vi "Nodos_Propiedad_Act02.vi"() -> ()   [LabVIEW 2020]
panel:
  in  "stop":bool
  out "String":string
  out "No. Muestreos":i32
  in  "Límite Muestreo":i32
  in  "Límite superior":dbl
  in  "Tiempo de muestreo":dbl
  out "Fuera de rango":bool
  out "Temperatura":cluster{dbl, "Límite superior":dbl}(graph)
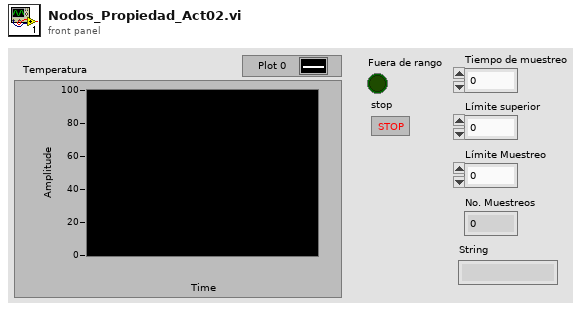
[diagram p1: front panel]
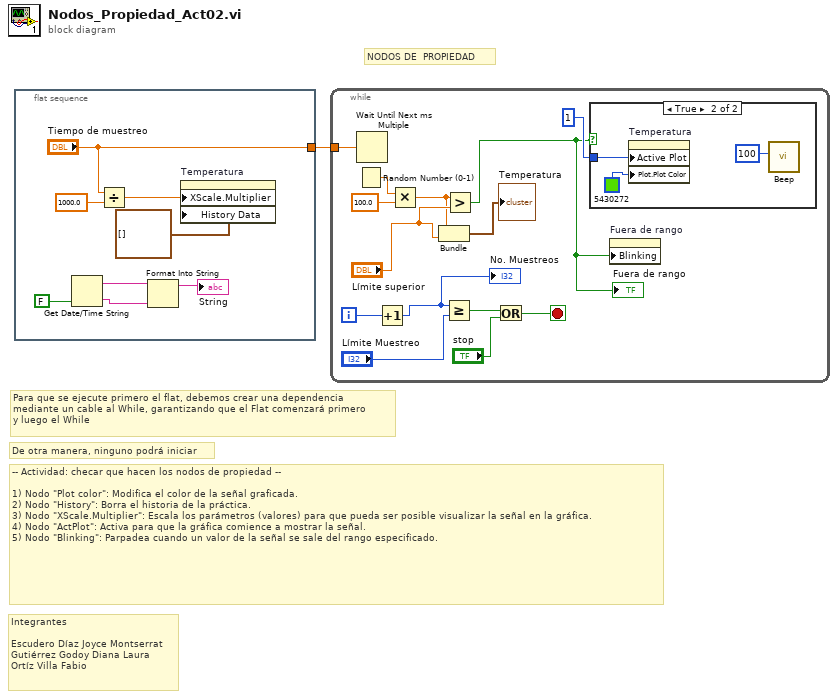
[diagram p0: block diagram]
diagram:
  # "Integrantes\n\nEscudero Díaz Joyce Montserrat\nGutiérrez Godoy Diana Laura\nOrtíz Villa Fabio"
  # "NODOS DE  PROPIEDAD"
  # "-- Actividad: checar que hacen los nodos de propiedad --\n\n1) Nodo \"Plot color\": Modifica el color de la señal graficada.\n2) Nodo \"History\": Borra el historia de la práctica.\n3) Nodo \"XScale.Multiplier\": Escala los parámetros (valores) para que pueda ser posible visualizar la señal en la gráfica.\n4) Nodo \"ActPlot\": Activa para que la gráfica comience a mostrar la señal.\n5) Nodo \"Blinking\": Parpadea cuando un valor de la señal se sale del rango especificado."
  # "De otra manera, ninguno podrá iniciar"
  # "Para que se ejecute primero el flat, debemos crear una dependencia\nmediante un cable al While, garantizando que el Flat comenzará primero\ny luego el While"
  n1 = flat-sequence {
    tunnel: ["Tiempo de muestreo"] -> w1
    frame #0 {
      n2 = Get Date/Time String(want seconds? (F)=FALSE) -> (date string=w8:string, time string=w7:string)  [unwired: 2 in]
      n3 = Divide(x="Tiempo de muestreo", y=1000.0) -> (x/y=w4:dbl)
      n4 = Format Into String(initial string=w8, w7) -> (resulting string=→"String":string)  [unwired: 2 in, 1 out]
      n5 = property on="Temperatura" class="WFChart (strict)"("XScale.Multiplier"=w4, "History Data"=cluster{dbl, "Límite superior":dbl}[] []) -> ()  [unwired: 2 in, 2 out]
    }
  }
  n6 = while {
    tunnel: w1 -> [w23]
    i -> [w18]
    stop <- w16 stop-if-true
    n7 = Random Number (0-1)() -> (number: 0 to 1=w21:dbl)
    n8 = Wait Until Next ms Multiple(millisecond multiple=w23) -> ()  [unwired: 1 out]
    n9 = Increment(x=w18) -> (x+1=w15:i32)
    "No. Muestreos" <- w15
    n10 = Multiply(x=w21, y=100.0) -> (x*y=w19:dbl)
    n11 = Bundle(w19, "Límite superior"="Límite superior") -> (→"Temperatura":cluster{dbl, "Límite superior":dbl})  [unwired: 1 in]
    n12 = Greater Or Equal?(x=w15, y="Límite Muestreo") -> (x >= y?=w17:bool)
    n13 = Greater?(x=w19, y="Límite superior") -> (0:w10:bool)
    "Fuera de rango" <- w10
    n14 = Or(x=w17, y="stop") -> (x .or. y?=w16:bool)
    n15 = case shown="True" w10 {
      tunnel: 1 -> [_ w26]
      frame False {
      }
      frame True {
        n16 = property on="Temperatura" class="WFChart (strict)"("Active Plot"=w26, "Plot.Plot Color"=u32 5430272) -> ()  [unwired: 2 in, 2 out]
        n17 = call <vilib>:"Beep.vi"("duration (msec)"=u32 100) -> ()  [unwired: 11 in]
      }
    }
    n18 = property on="Fuera de rango" class="Bool (strict)"("Blinking"=w10) -> ()  [unwired: 2 in, 2 out]
  }
